vi "Calibrate.vi"(0 "Array 2":dbl[][](array[numeric]), 1 "Starting Wavelength":dbl, 3 "Threshold":dbl, 4 "Wavelength/Step":dbl, 5 "End Blue":dbl=260.0, 6 "M0":bool, 7 "End Green":dbl, 8 "STOP REF":refnum<vi>, 9 "M1":bool) -> (2 "appended array":dbl[](array[numeric]))   [LabVIEW 2021]
panel:
  out "Wavelength/Step":dbl
  out "Start Wavelength":dbl
  in  "stop 2":bool
  in  "Blue Wavelength":dbl=442.8
  in  "Red Wavelength":dbl=685.1
  in  "Green Wavelength":dbl=532.34
  in  "stop":bool
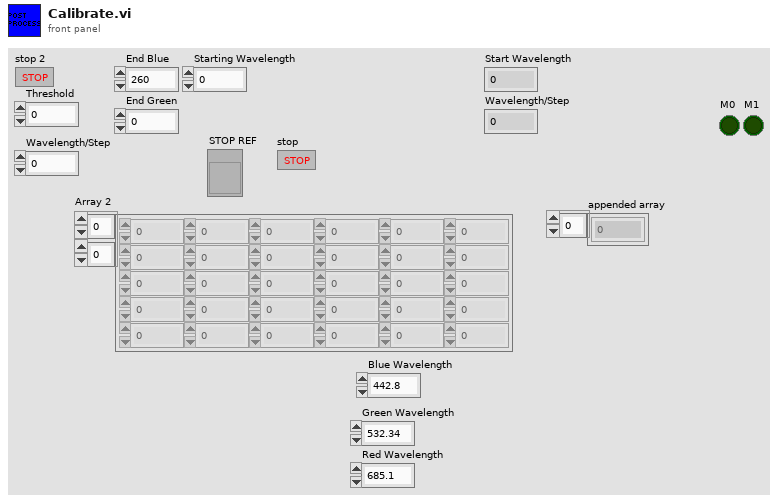
[diagram p1: front panel]
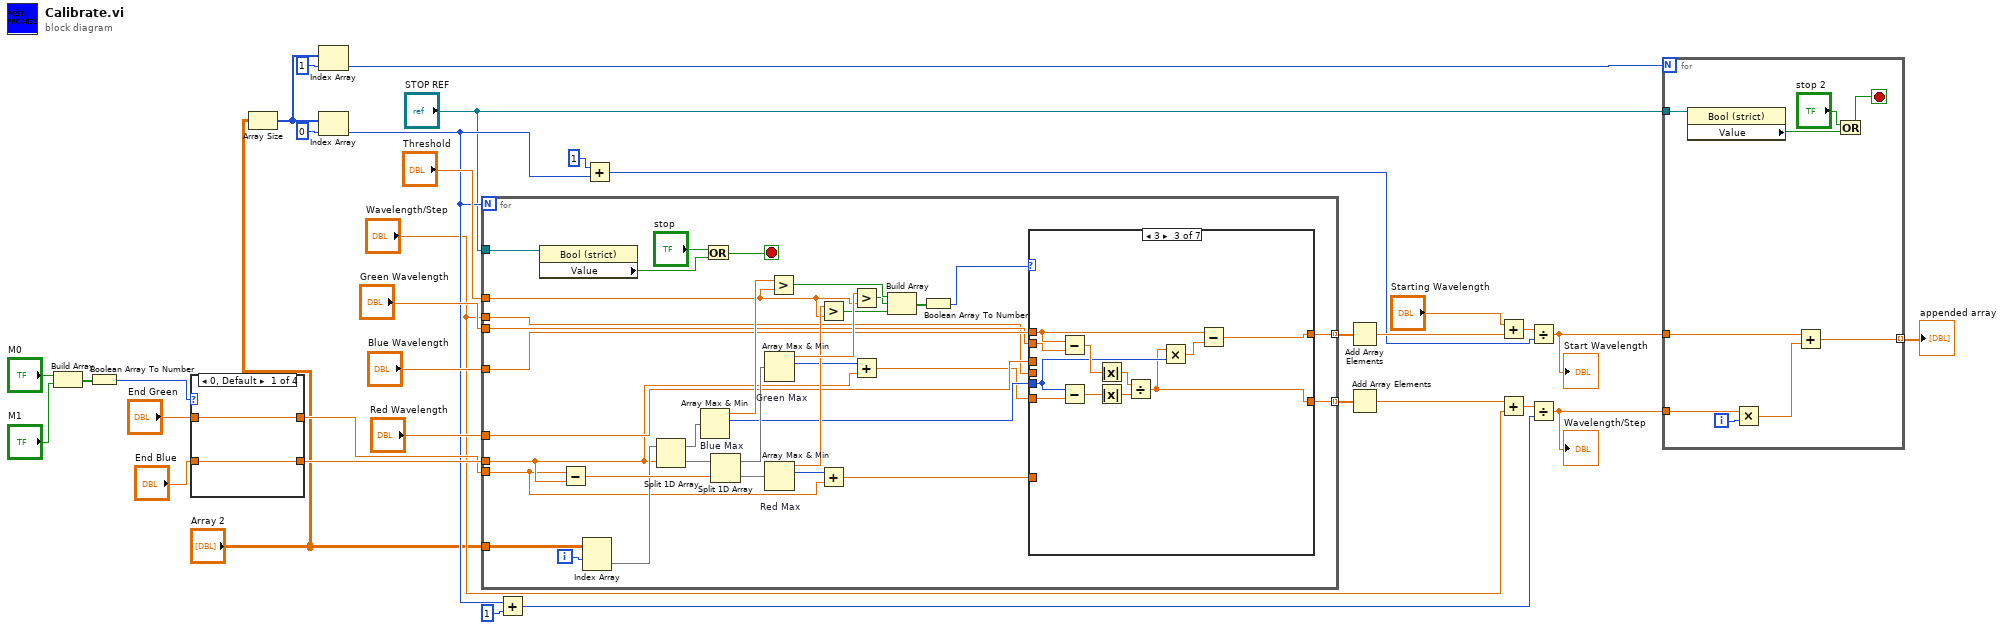
[diagram p0: block diagram]
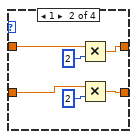
[diagram p2: hidden frame]
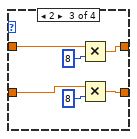
[diagram p3: hidden frame]
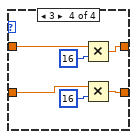
[diagram p4: hidden frame]
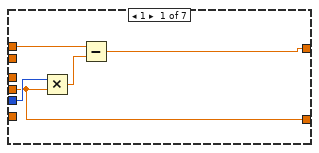
[diagram p5: hidden frame]
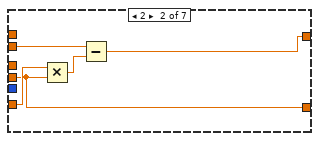
[diagram p6: hidden frame]
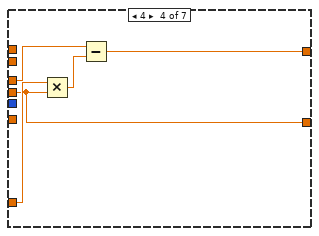
[diagram p7: hidden frame]
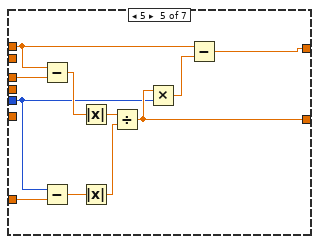
[diagram p8: hidden frame]
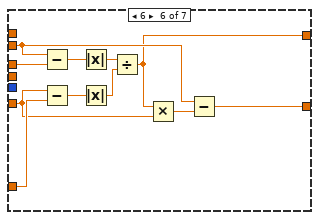
[diagram p9: hidden frame]
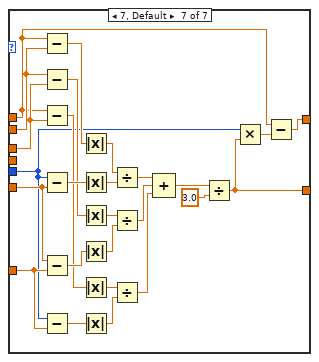
[diagram p10: hidden frame]
diagram:
  n1 = Build Array("M0", "M1") -> (w24:bool[])
  n2 = Boolean Array To Number(Boolean array=w24) -> (number=w23:u32)
  n3 = case shown="0, Default" w23 {
    tunnel: "End Blue" -> [w36 w40 w47 w53]
    tunnel: [w36 w39 w46 w52] -> w21
    tunnel: "End Green" -> [w35 w38 w44 w50]
    tunnel: [w35 w37 w43 w49] -> w19
    frame 0, Default {
    }
    frame 1 {
      n4 = Multiply(x=w38, y=2) -> (x*y=w37:dbl)
      n5 = Multiply(x=w40, y=2) -> (x*y=w39:dbl)
    }
    frame 2 {
      n6 = Multiply(x=w44, y=8) -> (x*y=w43:dbl)
      n7 = Multiply(x=w47, y=8) -> (x*y=w46:dbl)
    }
    frame 3 {
      n8 = Multiply(x=w50, y=16) -> (x*y=w49:dbl)
      n9 = Multiply(x=w53, y=16) -> (x*y=w52:dbl)
    }
  }
  n10 = Array Size(array="Array 2") -> (size(s)=w2:i32[])
  n11 = Index Array(array=w2, index=1) -> (element=w1:i32)
  n12 = Index Array(array=w2, index=0) -> (element=w10:i32)
  n13 = for {
    N: w10 -> [_]
    tunnel: "Array 2" -> [w88]
    tunnel: w21 -> [w59]
    tunnel: w19 -> [w56]
    tunnel: "Blue Wavelength" -> [w69]
    tunnel: "Green Wavelength" -> [w68]
    tunnel: "Red Wavelength" -> [w67]
    tunnel: [w66] -> w28 mode=indexing
    tunnel: [w65] -> w27 mode=indexing
    tunnel: "STOP REF" -> [w64]
    tunnel: "Threshold" -> [w63]
    tunnel: "Wavelength/Step" -> [w62]
    i -> [w87]
    stop <- w71 stop-if-true
    n14 = property class="Bool (strict)"(reference=w64) -> ("Value"=w72:bool)  [unwired: 1 in, 2 out]
    n15 = Subtract(x=w56, y=w59) -> (x-y=w85:dbl)
    n16 = Index Array(array=w88, index (row)=w87) -> (element=w61:dbl[])  [unwired: 1 in]
    n17 = Split 1D Array(array=w61, index=w59) -> (first subarray=w84:dbl[], second subarray=w86:dbl[])
    n18 = Array Max & Min "Blue Max"(array=w84) -> (max value=w83:dbl, max index (indices)=w70:i32)  [unwired: 2 out]
    n19 = Or(x="stop", y=w72) -> (x .or. y?=w71:bool)
    n20 = Split 1D Array(array=w86, index=w85) -> (first subarray=w81:dbl[], second subarray=w78:dbl[])
    n21 = Array Max & Min "Green Max"(array=w81) -> (max value=w80:dbl, max index (indices)=w60:i32)  [unwired: 2 out]
    n22 = Array Max & Min "Red Max"(array=w78) -> (max value=w77:dbl, max index (indices)=w57:i32)  [unwired: 2 out]
    n23 = Greater?(x=w83, y=w63) -> (0:w82:bool)
    n24 = Greater?(x=w77, y=w63) -> (0:w76:bool)
    n25 = Add(x=w57, y=w56) -> (x+y=w55:dbl)
    n26 = Greater?(x=w80, y=w63) -> (0:w79:bool)
    n27 = Add(x=w60, y=w59) -> (x+y=w58:dbl)
    n28 = Build Array(w82, w79, w76) -> (w75:bool[])
    n29 = Boolean Array To Number(Boolean array=w75) -> (number=w74:u32)
    n30 = case shown="3" w74 {
      tunnel: w70 -> [w91 _ w101 _ w116 _ w140]
      tunnel: w58 -> [_ w96 w107 _ _ w128 w162]
      tunnel: w55 -> [_ _ _ w111 w119 w131 w161]
      tunnel: w69 -> [w93 _ w102 _ w115 _ w139]
      tunnel: w68 -> [_ w95 w106 _ _ w129 w156]
      tunnel: w67 -> [_ _ _ w112 w120 w130 w155]
      tunnel: [w89 w94 w100 w110 w117 w126 w141] -> w66
      tunnel: [w90 w97 w99 w113 w118 w127 w137] -> w65
      tunnel: w62 -> [w89 w94 _ w110 _ _ _]
      frame 1 {
        n31 = Multiply(x=w91, y=w89) -> (x*y=w92:dbl)
        n32 = Subtract(x=w93, y=w92) -> (x-y=w90:dbl)
      }
      frame 2 {
        n33 = Multiply(x=w96, y=w94) -> (x*y=w98:dbl)
        n34 = Subtract(x=w95, y=w98) -> (x-y=w97:dbl)
      }
      frame 3 {
        n35 = Subtract(x=w102, y=w106) -> (x-y=w109:dbl)
        n36 = Subtract(x=w101, y=w107) -> (x-y=w108:dbl)
        n37 = Absolute Value(x=w109) -> (abs(x)=w105:dbl)
        n38 = Absolute Value(x=w108) -> (abs(x)=w104:dbl)
        n39 = Divide(x=w105, y=w104) -> (x/y=w100:dbl)
        n40 = Multiply(x=w100, y=w101) -> (x*y=w103:dbl)
        n41 = Subtract(x=w102, y=w103) -> (x-y=w99:dbl)
      }
      frame 4 {
        n42 = Multiply(x=w111, y=w110) -> (x*y=w114:dbl)
        n43 = Subtract(x=w112, y=w114) -> (x-y=w113:dbl)
      }
      frame 5 {
        n44 = Subtract(x=w115, y=w120) -> (x-y=w125:dbl)
        n45 = Subtract(x=w116, y=w119) -> (x-y=w124:dbl)
        n46 = Absolute Value(x=w125) -> (abs(x)=w123:dbl)
        n47 = Absolute Value(x=w124) -> (abs(x)=w122:dbl)
        n48 = Divide(x=w123, y=w122) -> (x/y=w117:dbl)
        n49 = Multiply(x=w117, y=w116) -> (x*y=w121:dbl)
        n50 = Subtract(x=w115, y=w121) -> (x-y=w118:dbl)
      }
      frame 6 {
        n51 = Subtract(x=w129, y=w130) -> (x-y=w132:dbl)
        n52 = Subtract(x=w128, y=w131) -> (x-y=w133:dbl)
        n53 = Absolute Value(x=w132) -> (abs(x)=w134:dbl)
        n54 = Absolute Value(x=w133) -> (abs(x)=w135:dbl)
        n55 = Divide(x=w134, y=w135) -> (x/y=w127:dbl)
        n56 = Multiply(x=w127, y=w128) -> (x*y=w136:dbl)
        n57 = Subtract(x=w129, y=w136) -> (x-y=w126:dbl)
      }
      frame 7, Default {
        n58 = Subtract(x=w139, y=w156) -> (x-y=w157:dbl)
        n59 = Subtract(x=w156, y=w155) -> (x-y=w154:dbl)
        n60 = Subtract(x=w139, y=w155) -> (x-y=w153:dbl)
        n61 = Subtract(x=w140, y=w162) -> (x-y=w160:dbl)
        n62 = Subtract(x=w162, y=w161) -> (x-y=w158:dbl)
        n63 = Subtract(x=w140, y=w161) -> (x-y=w159:dbl)
        n64 = Absolute Value(x=w157) -> (abs(x)=w149:dbl)
        n65 = Absolute Value(x=w160) -> (abs(x)=w152:dbl)
        n66 = Absolute Value(x=w154) -> (abs(x)=w148:dbl)
        n67 = Absolute Value(x=w158) -> (abs(x)=w151:dbl)
        n68 = Absolute Value(x=w153) -> (abs(x)=w147:dbl)
        n69 = Absolute Value(x=w159) -> (abs(x)=w150:dbl)
        n70 = Divide(x=w149, y=w152) -> (x/y=w146:dbl)
        n71 = Divide(x=w148, y=w151) -> (x/y=w145:dbl)
        n72 = Divide(x=w147, y=w150) -> (x/y=w144:dbl)
        n73 = Compound Arithmetic op=ADD(w146, w145, w144) -> (w143:dbl)
        n74 = Divide(x=w143, y=3.0) -> (x/y=w141:dbl)
        n75 = Multiply(x=w140, y=w141) -> (x*y=w138:dbl)
        n76 = Subtract(x=w139, y=w138) -> (x-y=w137:dbl)
      }
    }
  }
  n77 = Add(x=w10, y=1) -> (x+y=w13:i32)
  n78 = Add(x=1, y=w10) -> (x+y=w11:i32)
  n79 = Add Array Elements(numeric array=w27) -> (sum=w17:dbl)
  n80 = Add Array Elements(numeric array=w28) -> (sum=w16:dbl)
  n81 = Add(x="Starting Wavelength", y=w17) -> (x+y=w15:dbl)
  n82 = Add(x=w16, y="Wavelength/Step") -> (x+y=w7:dbl)
  n83 = Divide(x=w15, y=w11) -> (x/y=w5:dbl)
  "Start Wavelength" <- w5
  n84 = Divide(x=w7, y=w13) -> (x/y=w6:dbl)
  "Wavelength/Step" <- w6
  n85 = for {
    N: w1 -> [_]
    tunnel: [w164] -> w32 mode=indexing
    tunnel: w6 -> [w168]
    tunnel: w5 -> [w166]
    tunnel: "STOP REF" -> [w163]
    i -> [w167]
    stop <- w169 stop-if-true
    n86 = property class="Bool (strict)"(reference=w163) -> ("Value"=w170:bool)  [unwired: 1 in, 2 out]
    n87 = Multiply(x=w168, y=w167) -> (x*y=w165:dbl)
    n88 = Add(x=w166, y=w165) -> (x+y=w164:dbl)
    n89 = Or(x="stop 2", y=w170) -> (x .or. y?=w169:bool)
  }
  "appended array" <- w32
